vi "ReadRegister.vi"(5 "Address":u8, 7 "Bus":u8 format="%.0x", 8 "error in (no error)":errorcluster, 10 "Register":T1, 11 "VISA Refnum in":refnum<visa-resource-name>) -> (0 "error out":errorcluster, 2 "Numeric":i16, 3 "VISA Refnum out":refnum<visa-resource-name>)   [LabVIEW 2024]
uses:
  Register.ctl
  Driver/CTIPicoVISA.lvlib
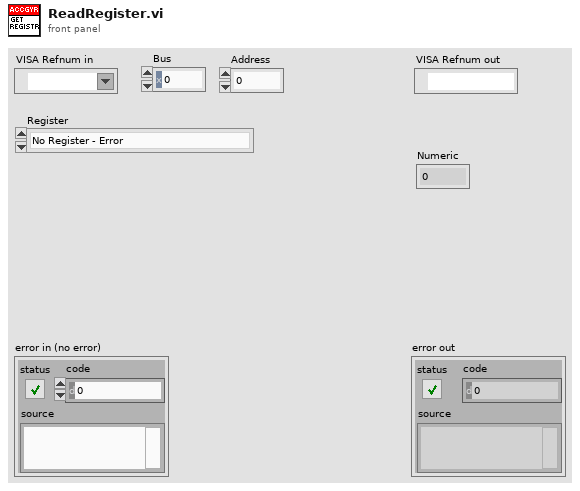
[diagram p1: front panel]
types:
  T1 = typedef "Register.ctl" = enum16{"No Register - Error", "D6D_SRC", "STATUS_REG", "OUT_TEMP_L", "OUT_TEMP_H", "OUTX_L_G", "OUTX_H_G", "OUTY_L_G", "OUTY_H_G", "OUTZ_L_G", "OUTZ_H_G", "OUTX_L_XL", "OUTX_H_XL", "OUTY_L_XL", "OUTY_H_XL", "OUTZ_L_XL", "OUTZ_H_XL", "SENSORHUB1_REG", "SENSORHUB2_REG", "SENSORHUB3_REG", "SENSORHUB4_REG", "SENSORHUB5_REG", "SENSORHUB6_REG", "SENSORHUB7_REG", "SENSORHUB8_REG", "SENSORHUB9_REG", "SENSORHUB10_REG", "SENSORHUB11_REG", "SENSORHUB12_REG"}
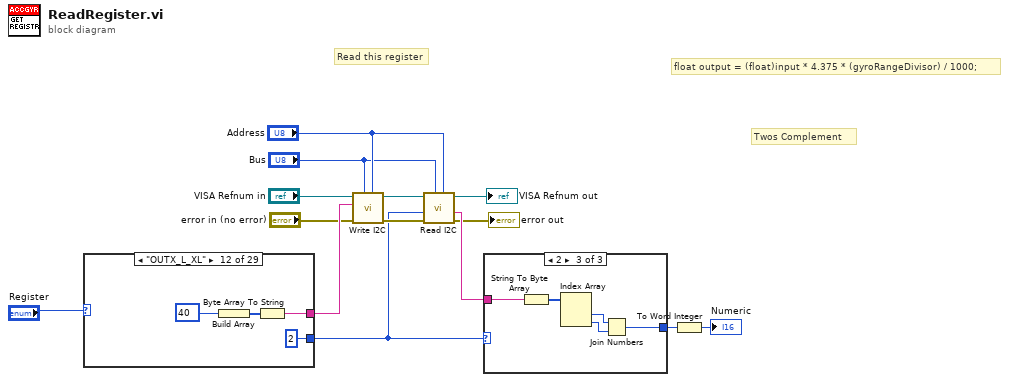
[diagram p0: block diagram]
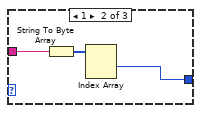
[diagram p3: hidden frame]
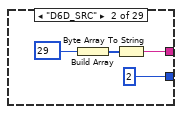
[diagram p5: hidden frame]
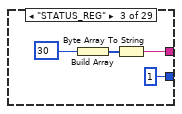
[diagram p6: hidden frame]
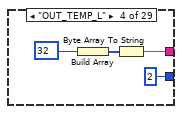
[diagram p7: hidden frame]
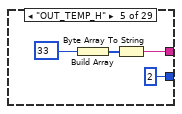
[diagram p8: hidden frame]
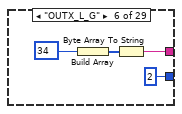
[diagram p9: hidden frame]
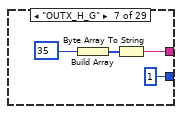
[diagram p10: hidden frame]
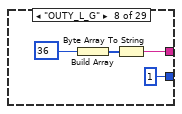
[diagram p11: hidden frame]
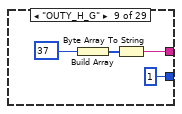
[diagram p12: hidden frame]
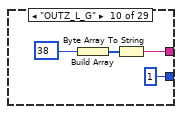
[diagram p13: hidden frame]
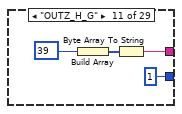
[diagram p14: hidden frame]
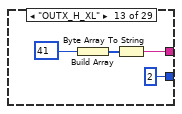
[diagram p15: hidden frame]
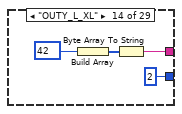
[diagram p16: hidden frame]
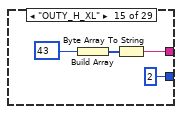
[diagram p17: hidden frame]
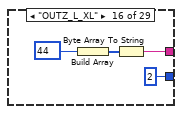
[diagram p18: hidden frame]
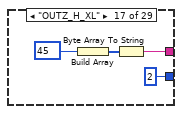
[diagram p19: hidden frame]
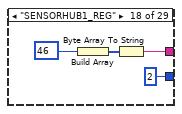
[diagram p20: hidden frame]
diagram:
  # "Twos Complement"
  # "float output = (float)input * 4.375 * (gyroRangeDivisor) / 1000;"
  # "Read this register"
  n1 = case shown="\"OUTX_L_XL\"" "Register" {
    tunnel: [_ w18 w22 w26 w30 w34 w38 w42 w46 w50 w54 w58 w62 w66 w70 w74 w78 w82 w86 w90 w94 w98 w102 w106 w110 w114 w118 w122 w126] -> w11
    tunnel: [_ u8 2 ("Len") u8 1 ("Len") u8 2 ("Len") u8 2 ("Len") u8 2 ("Len") u8 1 ("Len") u8 1 ("Len") u8 1 ("Len") u8 1 ("Len") u8 1 ("Len") u8 2 ("Len") u8 2 ("Len") u8 2 ("Len") u8 2 ("Len") u8 2 ("Len") u8 2 ("Len") u8 2 ("Len") u8 2 ("Len") u8 1 ("Len") u8 1 ("Len") u8 1 ("Len") u8 1 ("Len") u8 1 ("Len") u8 1 ("Len") u8 1 ("Len") u8 1 ("Len") u8 1 ("Len") u8 1 ("Len")] -> w2
    frame "No Register - Error", Default {
    }
    frame "D6D_SRC" {
      n2 = Build Array(u8 29 ("GYRO_OUTX_L_G")) -> (w16:u8[])
      n3 = Byte Array To String(unsigned byte array=w16) -> (string=w18:string)
    }
    frame "STATUS_REG" {
      n4 = Build Array(u8 30 ("GYRO_OUTX_L_G")) -> (w20:u8[])
      n5 = Byte Array To String(unsigned byte array=w20) -> (string=w22:string)
    }
    frame "OUT_TEMP_L" {
      n6 = Build Array(u8 32 ("GYRO_OUTX_L_G")) -> (w24:u8[])
      n7 = Byte Array To String(unsigned byte array=w24) -> (string=w26:string)
    }
    frame "OUT_TEMP_H" {
      n8 = Build Array(u8 33 ("GYRO_OUTX_L_G")) -> (w28:u8[])
      n9 = Byte Array To String(unsigned byte array=w28) -> (string=w30:string)
    }
    frame "OUTX_L_G" {
      n10 = Build Array(u8 34 ("GYRO_OUTX_L_G")) -> (w32:u8[])
      n11 = Byte Array To String(unsigned byte array=w32) -> (string=w34:string)
    }
    frame "OUTX_H_G" {
      n12 = Build Array(u8 35 ("GYRO_OUTX_L_G")) -> (w36:u8[])
      n13 = Byte Array To String(unsigned byte array=w36) -> (string=w38:string)
    }
    frame "OUTY_L_G" {
      n14 = Build Array(u8 36 ("GYRO_OUTX_L_G")) -> (w40:u8[])
      n15 = Byte Array To String(unsigned byte array=w40) -> (string=w42:string)
    }
    frame "OUTY_H_G" {
      n16 = Build Array(u8 37 ("GYRO_OUTX_L_G")) -> (w44:u8[])
      n17 = Byte Array To String(unsigned byte array=w44) -> (string=w46:string)
    }
    frame "OUTZ_L_G" {
      n18 = Build Array(u8 38 ("GYRO_OUTX_L_G")) -> (w48:u8[])
      n19 = Byte Array To String(unsigned byte array=w48) -> (string=w50:string)
    }
    frame "OUTZ_H_G" {
      n20 = Build Array(u8 39 ("GYRO_OUTX_L_G")) -> (w52:u8[])
      n21 = Byte Array To String(unsigned byte array=w52) -> (string=w54:string)
    }
    frame "OUTX_L_XL" {
      n22 = Build Array(u8 40 ("GYRO_OUTX_L_G")) -> (w56:u8[])
      n23 = Byte Array To String(unsigned byte array=w56) -> (string=w58:string)
    }
    frame "OUTX_H_XL" {
      n24 = Build Array(u8 41 ("GYRO_OUTX_L_G")) -> (w60:u8[])
      n25 = Byte Array To String(unsigned byte array=w60) -> (string=w62:string)
    }
    frame "OUTY_L_XL" {
      n26 = Build Array(u8 42 ("GYRO_OUTX_L_G")) -> (w64:u8[])
      n27 = Byte Array To String(unsigned byte array=w64) -> (string=w66:string)
    }
    frame "OUTY_H_XL" {
      n28 = Build Array(u8 43 ("GYRO_OUTX_L_G")) -> (w68:u8[])
      n29 = Byte Array To String(unsigned byte array=w68) -> (string=w70:string)
    }
    frame "OUTZ_L_XL" {
      n30 = Build Array(u8 44 ("GYRO_OUTX_L_G")) -> (w72:u8[])
      n31 = Byte Array To String(unsigned byte array=w72) -> (string=w74:string)
    }
    frame "OUTZ_H_XL" {
      n32 = Build Array(u8 45 ("GYRO_OUTX_L_G")) -> (w76:u8[])
      n33 = Byte Array To String(unsigned byte array=w76) -> (string=w78:string)
    }
    frame "SENSORHUB1_REG" {
      n34 = Build Array(u8 46 ("GYRO_OUTX_L_G")) -> (w80:u8[])
      n35 = Byte Array To String(unsigned byte array=w80) -> (string=w82:string)
    }
    frame "SENSORHUB2_REG" {
      n36 = Build Array(u8 47 ("GYRO_OUTX_L_G")) -> (w84:u8[])
      n37 = Byte Array To String(unsigned byte array=w84) -> (string=w86:string)
    }
    frame "SENSORHUB3_REG" {
      n38 = Build Array(u8 48 ("GYRO_OUTX_L_G")) -> (w88:u8[])
      n39 = Byte Array To String(unsigned byte array=w88) -> (string=w90:string)
    }
    frame "SENSORHUB4_REG" {
      n40 = Build Array(u8 49 ("GYRO_OUTX_L_G")) -> (w92:u8[])
      n41 = Byte Array To String(unsigned byte array=w92) -> (string=w94:string)
    }
    frame "SENSORHUB5_REG" {
      n42 = Build Array(u8 50 ("GYRO_OUTX_L_G")) -> (w96:u8[])
      n43 = Byte Array To String(unsigned byte array=w96) -> (string=w98:string)
    }
    frame "SENSORHUB6_REG" {
      n44 = Build Array(u8 51 ("GYRO_OUTX_L_G")) -> (w100:u8[])
      n45 = Byte Array To String(unsigned byte array=w100) -> (string=w102:string)
    }
    frame "SENSORHUB7_REG" {
      n46 = Build Array(u8 52 ("GYRO_OUTX_L_G")) -> (w104:u8[])
      n47 = Byte Array To String(unsigned byte array=w104) -> (string=w106:string)
    }
    frame "SENSORHUB8_REG" {
      n48 = Build Array(u8 53 ("GYRO_OUTX_L_G")) -> (w108:u8[])
      n49 = Byte Array To String(unsigned byte array=w108) -> (string=w110:string)
    }
    frame "SENSORHUB9_REG" {
      n50 = Build Array(u8 54 ("GYRO_OUTX_L_G")) -> (w112:u8[])
      n51 = Byte Array To String(unsigned byte array=w112) -> (string=w114:string)
    }
    frame "SENSORHUB10_REG" {
      n52 = Build Array(u8 55 ("GYRO_OUTX_L_G")) -> (w116:u8[])
      n53 = Byte Array To String(unsigned byte array=w116) -> (string=w118:string)
    }
    frame "SENSORHUB11_REG" {
      n54 = Build Array(u8 56 ("GYRO_OUTX_L_G")) -> (w120:u8[])
      n55 = Byte Array To String(unsigned byte array=w120) -> (string=w122:string)
    }
    frame "SENSORHUB12_REG" {
      n56 = Build Array(u8 57 ("GYRO_OUTX_L_G")) -> (w124:u8[])
      n57 = Byte Array To String(unsigned byte array=w124) -> (string=w126:string)
    }
  }
  n58 = call "Write I2C.vi"("Address"="Address", "Bus"="Bus", "error in (no error)"="error in (no error)", "Data"=w11, "VISA resource name in"="VISA Refnum in") -> ("error out"=w7:errorcluster, "VISA resource name"=w8:refnum<visa-resource-name>)  [unwired: 5 in]
  n59 = call "Read I2C.vi"("Address"="Address", "Bus"="Bus", "error in (no error)"=w7, "Len"=w2, "VISA resource name in"=w8) -> ("error out"=→"error out":errorcluster, "Data"=w13:string, "VISA resource name"=→"VISA Refnum out":refnum<visa-resource-name>)  [unwired: 4 in]
  n60 = case shown="2" w2 {
    tunnel: [_ w127 w134] -> w14
    tunnel: w13 -> [_ w128 w132]
    frame 0, Default {
    }
    frame 1 {
      n61 = String To Byte Array(string=w128) -> (unsigned byte array=w129:u8[])
      n62 = Index Array(array=w129) -> (element #1=w127:u8)  [unwired: 2 in, 1 out]
    }
    frame 2 {
      n63 = String To Byte Array(string=w132) -> (unsigned byte array=w133:u8[])
      n64 = Index Array(array=w133) -> (element #1=w131:u8, element #2=w130:u8)  [unwired: 2 in]
      n65 = Join Numbers(hi=w131, lo=w130) -> ((hi.lo)=w134:u16)
    }
  }
  n66 = To Word Integer(number=w14) -> (16bit integer=→"Numeric":i16)
